vi "Parse Arguments.vi"(8 "error in (no error)":errorcluster, 9 "Args":string[](array[string]), 10 "Folder":path, 11 "InstallAction in":refnum<class "InstallAction.lvclass">) -> (0 "error out":errorcluster, 3 "InstallAction out":refnum<class "InstallAction.lvclass">)   [LabVIEW 2020, in "GPackTools.lvlib" / "InstallAction.lvclass"]
uses:
  InstallAction.lvclass
  InstallAction.lvclass/InstallAction.ctl
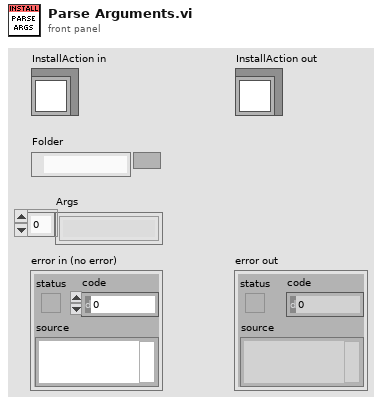
[diagram p1: front panel]
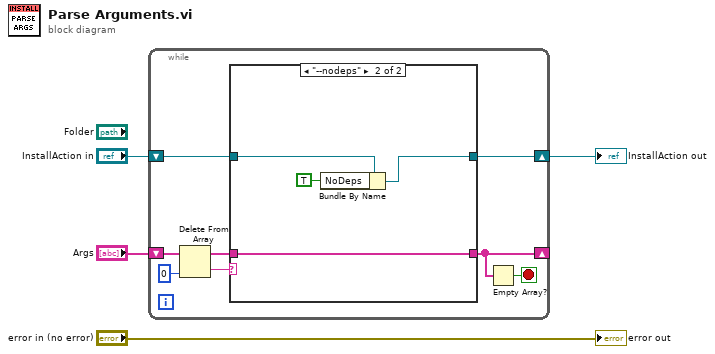
[diagram p0: block diagram]
diagram:
  n1 = while {
    shift-right: [w5] -> w2
    shift-left: "InstallAction in" -> [w6]
    shift-right: [w8] -> _
    shift-left: "Args" -> [w12]
    stop <- w7 stop-if-true
    n2 = Delete From Array(array=w12, index=0) -> (deleted portion=w10:string, array with subset deleted=w9:string[])  [unwired: 1 in]
    n3 = case shown="\"--nodeps\"" w10 {
      tunnel: w9 -> [w14 w18]
      tunnel: [w14 w18] -> w8
      tunnel: w6 -> [w13 w17]
      tunnel: [w13 w16] -> w5
      frame Default {
      }
      frame "--nodeps" {
        n4 = Bundle By Name(cluster=w17, "NoDeps"=TRUE) -> (w16:refnum<class "InstallAction.lvclass">)
      }
    }
    n5 = Empty Array?(array=w8) -> (empty?=w7:bool)
  }
  "InstallAction out" <- w2
  "error out" <- "error in (no error)"
